vi "AO-Freq.vi"(4 "GuiRef":T1, 5 "Slot":T3, 8 "error in":errorcluster, 9 "AMP":dbl, 10 "Freq":dbl, 11 "CH":string) -> (0 "error out":errorcluster)   [LabVIEW 2013]
uses:
  SystemCode/SysControl/Slot.ctl
  SystemCode/SysControl/Reference.ctl
  SystemCode/SysControl/TestItemsCTL.ctl
  SourceCode/GlobalValue.vi
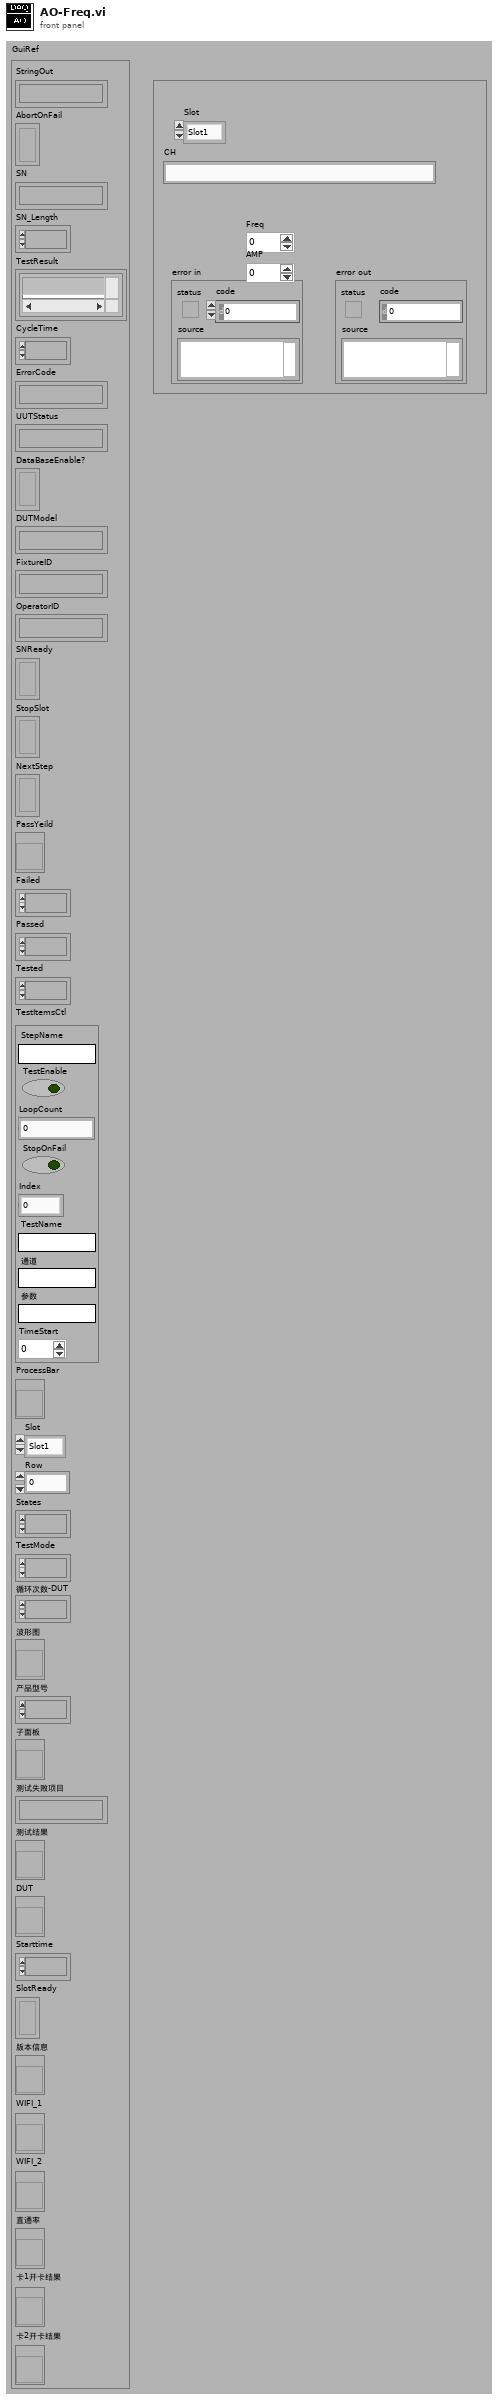
[diagram p1: front panel]
types:
  T1 = typedef "Reference.ctl" = cluster{"StringOut":refnum<vi>, "AbortOnFail":refnum<vi>, "SN":refnum<vi>, "SN_Length":refnum<vi>, "TestResult":refnum<vi>, "CycleTime":refnum<vi>, "ErrorCode":refnum<vi>, "UUTStatus":refnum<vi>, "DataBaseEnable?":refnum<vi>, "DUTModel":refnum<vi>, "FixtureID":refnum<vi>, "OperatorID":refnum<vi>, "SNReady":refnum<vi>, "StopSlot":refnum<vi>, "NextStep":refnum<vi>, "PassYeild":refnum<vi>, "Failed":refnum<vi>, "Passed":refnum<vi>, "Tested":refnum<vi>, "TestItemsCtl":T2, "ProcessBar":refnum<vi>, "Slot":T3, "Row":u32, "States":refnum<vi>, "TestMode":refnum<vi>, "循环次数-DUT":refnum<vi>, "波形图":refnum<vi>, "产品型号":refnum<vi>, "子面板":refnum<vi>, "测试失败项目":refnum<vi>, "测试结果":refnum<vi>, "DUT":refnum<vi>, "Starttime":refnum<vi>, "SlotReady":refnum<vi>, "版本信息":refnum<vi>, "WIFI_1":refnum<vi>, "WIFI_2":refnum<vi>, "直通率":refnum<vi>, "卡1开卡结果":refnum<vi>, "卡2开卡结果":refnum<vi>}
  T2 = typedef "TestItemsCTL.ctl" = cluster{"StepName":string, "TestEnable":bool, "LoopCount":i32, "StopOnFail":bool, "Index":u32, "TestName":string, "通道":string, "参数":string, "TimeStart":u32}
  T3 = typedef "Slot.ctl" = enum16{"Slot1", "Slot2", "Slot3", "Slot4"}
  T4 = typedef "DAQConfig.ctl" = cluster{"DIO":string[][], "AO":string[][], "AI":string[][]}
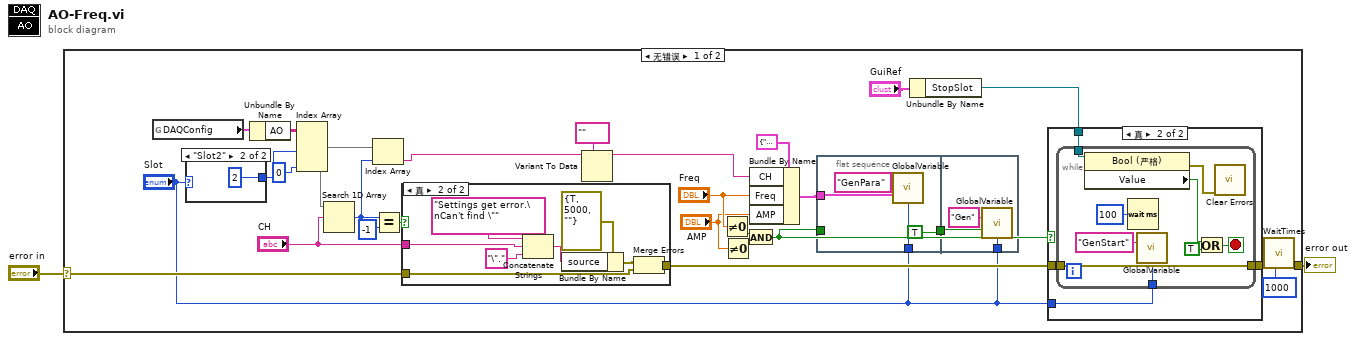
[diagram p0: block diagram]
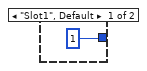
[diagram p2: hidden frame]
diagram:
  n1 = case shown="无错误" "error in" {
    selector: "error in" -> [w23 w64]
    tunnel: [w8 w64] -> w1
    frame No Error {
      n2 = global read "GlobalValue.vi" "DAQConfig"() -> (w11:T4)
      n3 = case shown="\"Slot2\"" "Slot" {
        tunnel: [1 ("索引 (行)") 2 ("索引 (行)")] -> w12
        frame "Slot1", Default {
        }
        frame "Slot2" {
        }
      }
      n4 = Unbundle By Name(w11) -> ("AO"=w31:string[][])
      n5 = Index Array(array=w31, index (col) #1=w12, index (col) #2=0 ("索引 (列)")) -> (element #1=w27:string[], element #2=w26:string[])  [unwired: 2 in]
      n6 = Search 1D Array(1D array=w26, element="CH") -> (index of element=w29:i32)  [unwired: 1 in]
      n7 = Index Array(array=w27, index=w29) -> (element=w21:string)
      n8 = Equal?(x=w29, y=-1) -> (x = y?=w25:bool)
      n9 = case shown="真" w25 {
        tunnel: w23 -> [w55 w59]
        tunnel: [w55 w58] -> w7
        tunnel: "CH" -> [_ w57]
        frame False {
        }
        frame True {
          n10 = Concatenate Strings("Settings get error.\nCan't find \"" ("message"), w57, "\"." ("string")) -> (w62:string)
          n11 = Bundle By Name(cluster=errorcluster {"status"=TRUE, "code"=5000, "source"=""} ("error in 1 (no error)"), "source"=w62) -> (w61:errorcluster)
          n12 = Merge Errors(w61, w59) -> (w58:errorcluster)
        }
      }
      n13 = Variant To Data(type=tag "" ("lines"), Variant=w21) -> (data=w20:tag)  [unwired: 1 in, 1 out]
      n14 = Not Equal To 0?(x="Freq") -> (x != 0?=w19:bool)
      n15 = Not Equal To 0?(x="AMP") -> (x != 0?=w18:bool)
      n16 = And(x=w19, y=w18) -> (x .and. y?=w6:bool)
      n17 = Bundle By Name(cluster=cluster{"CH":tag, "Freq":dbl, "AMP":dbl} {"CH"="Dev1/ao1", "Freq"=0.0, "AMP"=0.0} ("Paras 2"), "CH"=w20, "Freq"="Freq", "AMP"="AMP") -> (w4:cluster{"CH":tag, "Freq":dbl, "AMP":dbl})
      n18 = flat-sequence {
        tunnel: w6 -> [_]
        tunnel: [TRUE] -> w5
        tunnel: w4 -> [w34]
        tunnel: "Slot" -> [w33]
        tunnel: w5 -> [w37]
        tunnel: "Slot" -> [w36]
        frame #0 {
          n19 = call "GlobalVariable.vi"("Name"="GenPara", "ValueIn"=w34, "Slot"=w33) -> ()  [unwired: 9 in, 4 out]
        }
        frame #1 {
          n20 = call "GlobalVariable.vi"("Name"="Gen", "ValueIn"=w37, "Slot"=w36) -> ()  [unwired: 9 in, 4 out]
        }
      }
      n21 = Unbundle By Name("GuiRef") -> ("StopSlot"=w9:refnum<vi>)
      n22 = case shown="真" w6 {
        tunnel: w7 -> [w41 w45]
        tunnel: [w41 w44] -> w14
        tunnel: w9 -> [_ w43]
        tunnel: "Slot" -> [_ w42]
        frame False {
        }
        frame True {
          n23 = while {
            tunnel: w45 -> [w49]
            tunnel: [w49] -> w44
            tunnel: w43 -> [w53]
            tunnel: w42 -> [w48]
            stop <- w51 stop-if-true
            n24 = property class="Bool (严格)"(reference=w53) -> (error out=w46:errorcluster, "Value"=w52:bool)  [unwired: 1 in, 1 out]
            n25 = Wait (ms)(milliseconds to wait=u32 100 ("等待时间（毫秒）")) -> ()  [unwired: 1 out]
            n26 = call "GlobalVariable.vi"("Name"="GenStart", "Slot"=w48) -> ()  [unwired: 10 in, 4 out]
            n27 = Or(x=w52, y=TRUE) -> (x .or. y?=w51:bool)
            n28 = call <vilib>:"Clear Errors.vi"("error in (no error)"=w46) -> ()  [unwired: 6 in, 1 out]
          }
        }
      }
      n29 = call "WaitTimes.vi"("WaitTimes"=u32 1000, "error in (no error)"=w14) -> ("error out"=w8:errorcluster)  [unwired: 9 in]
    }
    frame Error {
    }
  }
  "error out" <- w1
